vi "testLaserComms_2.vi"() -> ()   [LabVIEW 2015]
uses:
  <vilib>/Instr/_visa.llb/VISA Configure Serial Port (Instr).vi
panel:
  out "concatenated string":string
  out "read buffer":string
  in  "laser power (mW)":dbl
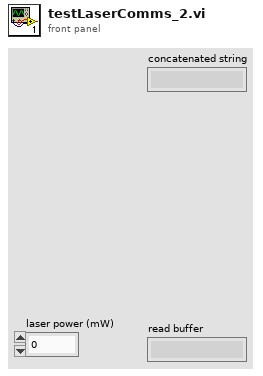
[diagram p1: front panel]
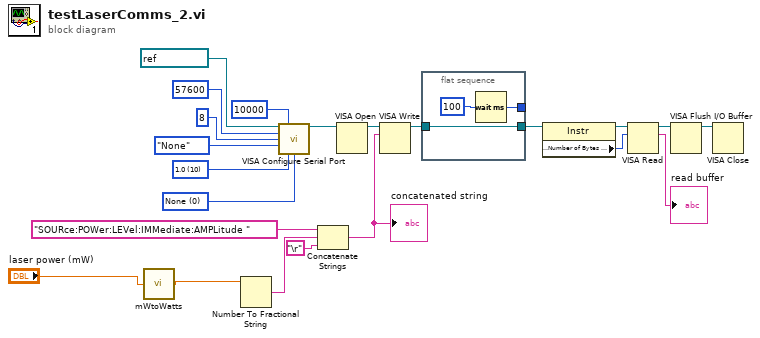
[diagram p0: block diagram]
diagram:
  w16 = u16 0 items=["None", "XON/XOFF", "RTS/CTS", "XON/XOFF & RTS/CTS", "DTR/DSR", "XON/XOFF & DTR/DSR"] ("flow control (0:none)")
  w17 = u16 10 items=["1.0"=10, "1.5"=15, "2.0"=20] ("stop bits (10: 1 bit)")
  n1 = call "mWtoWatts.vi"("mW"="laser power (mW)") -> ("W"=w1:dbl)
  n2 = Number To Fractional String(number=w1) -> (F-format string=w12:string)  [unwired: 3 in]
  n3 = call-poly "VISA Configure Serial Port"("VISA resource name"=refnum<visa-resource-name> "COM27", "timeout (10sec)"=u32 10000, "baud rate (9600)"=u32 57600, "data bits (8)"=u16 8, "parity (0:none)"=enum16{"None", "Odd", "Even", "Mark", "Space"}."None", "stop bits (10: 1 bit)"=w17, "flow control (0:none)"=w16) -> ("VISA resource name out"=w15:refnum<visa-resource-name>)  [unwired: 7 in, 1 out]
  n4 = Concatenate Strings("SOURce:POWer:LEVel:IMMediate:AMPLitude " ("string"), w12, "\r") -> (w10:string)
  "concatenated string" <- w10
  n5 = VISA Open(VISA resource name=w15) -> (VISA resource name=w14:refnum<visa-resource-name>)  [unwired: 4 in, 1 out]
  n6 = VISA Write(VISA resource name=w14, write buffer=w10) -> (VISA resource name out=w9:refnum<visa-resource-name>)  [unwired: 1 in, 2 out]
  n7 = flat-sequence {
    tunnel: w9 -> [w25]
    tunnel: [w25] -> w5
    tunnel: [w23] -> _
    frame #0 {
      n8 = Wait (ms)(milliseconds to wait=u32 100) -> (millisecond timer value=w23:u32)
    }
  }
  n9 = property class="Instr"(reference=w5) -> (reference out=w7:refnum<visa-resource-name>, "Serial Settings:Number of Bytes at Serial Port"=w6:u32)  [unwired: 1 in, 1 out]
  n10 = VISA Read(VISA resource name=w7, byte count=w6) -> (VISA resource name out=w8:refnum<visa-resource-name>, read buffer=→"read buffer":string)  [unwired: 1 in, 2 out]
  n11 = VISA Flush I/O Buffer(VISA resource name=w8) -> (VISA resource name out=w3:refnum<visa-resource-name>)  [unwired: 2 in, 1 out]
  n12 = VISA Close(VISA resource name=w3) -> ()  [unwired: 1 in, 1 out]
